vi "Auto Configure DAQ.vi"(8 "error in (no error)":errorcluster, 11 "LockinDAQ":refnum<class "LockinDAQ.lvclass">) -> (0 "error out":errorcluster, 2 "New Ch []":T1[](array[typedef]) {"AI.Coupling" items=["AC"=10045, "DC"=10050, "GND"=10066]}, 3 "LockinDAQ out":refnum<class "LockinDAQ.lvclass">)   [LabVIEW 2016, in "LockinDAQ.lvclass"]
uses:
  LockinDAQ.lvclass
  Typedefs/New Channel Cluster.ctl
  Typedefs/446xAI-enum.ctl
  Typedefs/AI.coupling-enum.ctl
  Typedefs/446xAO-enum.ctl
  Typedefs/AO.config-cluster.ctl
  Typedefs/DAQType-enum.ctl
  Typedefs/AI.config-cluster.ctl
  LockinDAQ.lvclass/LockinDAQ.ctl
  <resource>/objmgr/daqmx.rc
panel:
  # "Device"
  # "AI.Ch"
  # "AI.Range"
  # "AI.Coupling"
  # "AO.Ch"
  # "AO.Range"
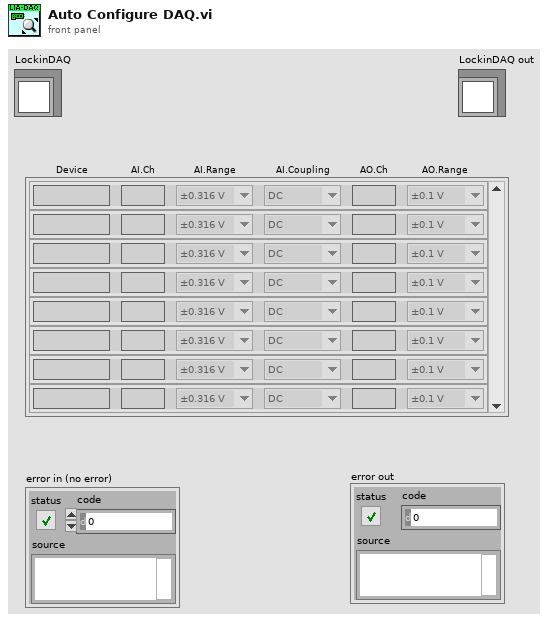
[diagram p1: front panel]
types:
  T1 = typedef "LockinDAQ.lvclass/New Channel Cluster.ctl" = cluster{"Device":string, "AI.Ch":string, "AI.Range":T2, "AI.Coupling":T3, "AO.Ch":string, "AO.Range":T4}
  T2 = typedef "LockinDAQ.lvclass/446xAI-enum.ctl" = enum16{"±0.316 V", "±1.00 V", "±3.16 V", "±10.0 V", "±31.6 V", "±42.4 V"}
  T3 = typedef "LockinDAQ.lvclass/AI.coupling-enum.ctl" = u16
  T4 = typedef "LockinDAQ.lvclass/446xAO-enum.ctl" = enum16{"±0.1 V", "±1.0 V", "±10.0 V"}
  T5 = typedef "LockinDAQ.lvclass/AI.config-cluster.ctl" = cluster{"AI.channels":tag, "AI.Coupling":T3, "AI.Range":T2, "input terminal configuration":i32, "DAQ Type":T6}
  T6 = typedef "LockinDAQ.lvclass/DAQType-enum.ctl" = enum16{"None", "USB 4431", "PXI 446x"}
  T7 = typedef "LockinDAQ.lvclass/AO.config-cluster.ctl" = cluster{"AO.channels":tag, "AO.Range":T4, "output terminal configuration":i32, "DAQ Type":T6}
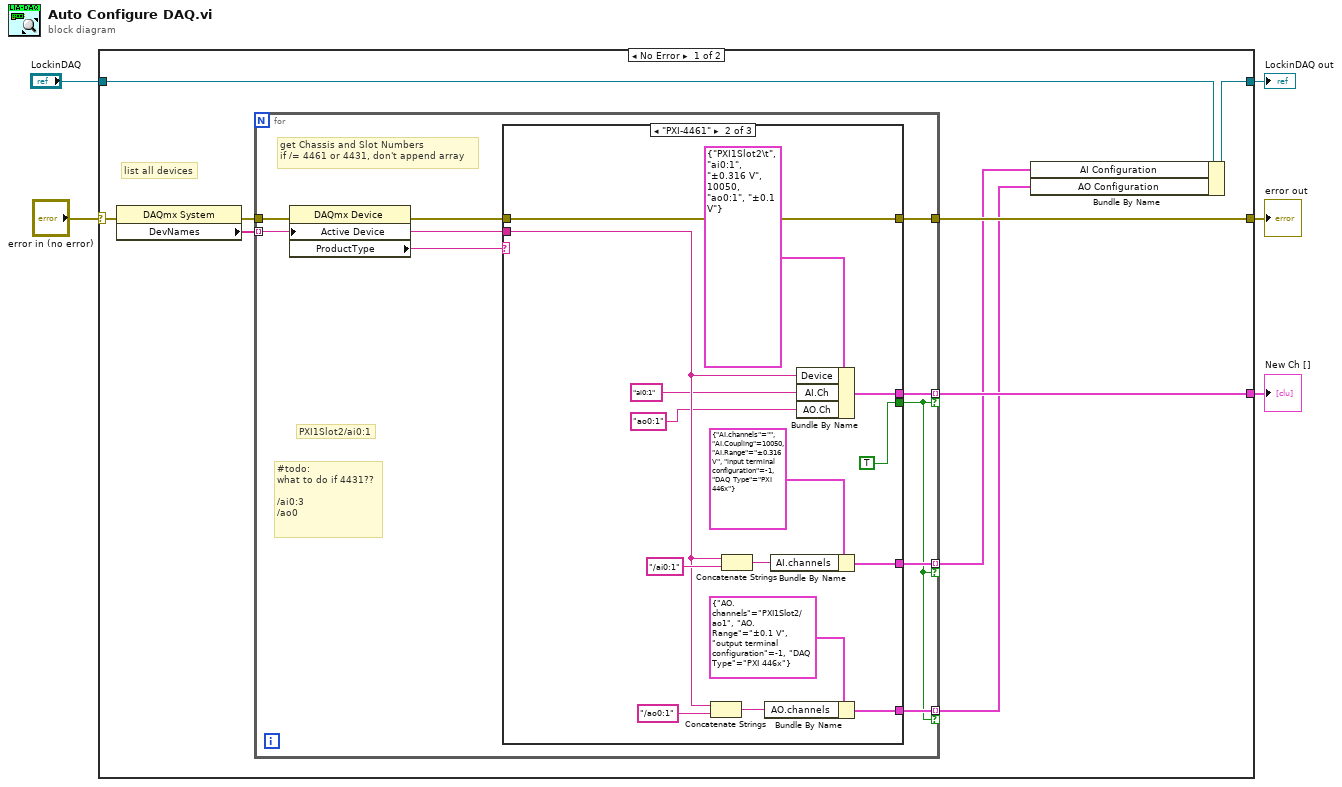
[diagram p0: block diagram]
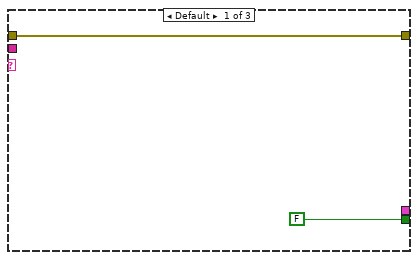
[diagram p2: hidden frame]
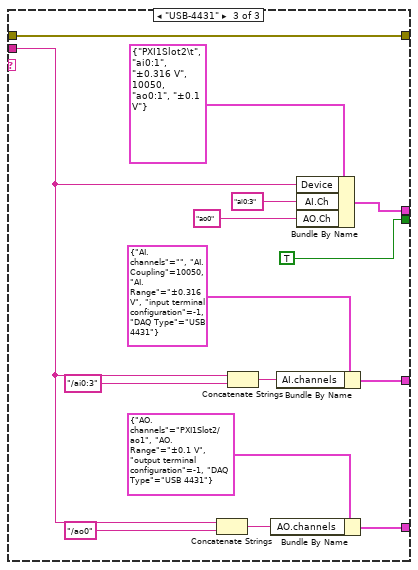
[diagram p3: hidden frame]
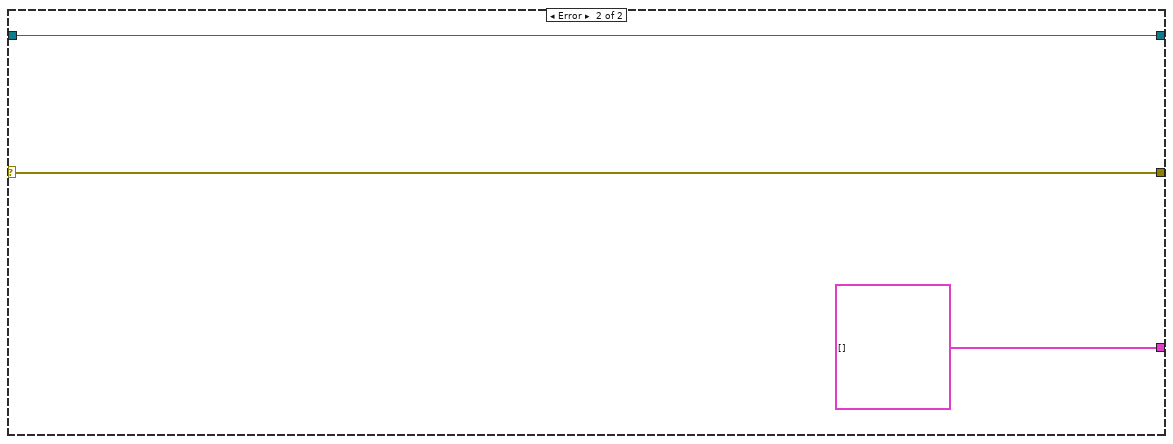
[diagram p4: hidden frame]
diagram:
  n1 = case shown="No Error" "error in (no error)" {
    selector: "error in (no error)" -> [w6 w57]
    tunnel: [w12 T1[] []] -> w5
    tunnel: [w11 w57] -> w4
    tunnel: "LockinDAQ" -> [w10 w58]
    tunnel: [w9 w58] -> w2
    frame No Error {
      # "list all devices"
      n2 = property class="DAQmx System"(error in=w6) -> (error out=w13:errorcluster, "DevNames"=w14:tag[])  [unwired: 1 in, 1 out]
      n3 = for {
        tunnel: w14 -> [w15] mode=indexing
        tunnel: w13 -> [w23]
        tunnel: [w22] -> w12 mode=indexing if=w18
        tunnel: [w16] -> w11
        tunnel: [w21] -> w8 mode=indexing if=w18
        tunnel: [w20] -> w7 mode=indexing if=w18
        # "#todo:\nwhat to do if 4431??\n\n/ai0:3\n/ao0"
        # "PXI1Slot2/ai0:1"
        # "get Chassis and Slot Numbers\nif /= 4461 or 4431, don't append array"
        n4 = property class="DAQmx Device"(error in=w23, "Active Device"=w15) -> (error out=w17:errorcluster, "ProductType"=w19:string)  [unwired: 1 in, 1 out]
        n5 = case shown="\"PXI-4461\"" w19 {
          tunnel: [_ w40 w55] -> w22
          tunnel: [_ w34 w49] -> w21
          tunnel: [_ w33 w48] -> w20
          tunnel: [FALSE TRUE TRUE] -> w18
          tunnel: w17 -> [w24 w29 w41]
          tunnel: [w24 w29 w41] -> w16
          tunnel: w15 -> [_ w28 w44]
          frame Default {
          }
          frame "PXI-4461" {
            n6 = Concatenate Strings(w28, "/ao0:1" ("string")) -> (w37:string)
            n7 = Concatenate Strings(w28, "/ai0:1" ("string")) -> (w31:string)
            n8 = Bundle By Name(cluster=T7 {"AO.channels"="PXI1Slot2/ao1", "AO.Range"=enum."±0.1 V", "output terminal configuration"=-1, "DAQ Type"=enum."PXI 446x"} ("AO.config"), "AO.channels"=w37) -> (w33:T7)
            n9 = Bundle By Name(cluster=T5 {"AI.channels"="", "AI.Coupling"=10050, "AI.Range"=enum."±0.316 V", "input terminal configuration"=-1, "DAQ Type"=enum."PXI 446x"} ("AI.Config"), "AI.channels"=w31) -> (w34:T5)
            n10 = Bundle By Name(cluster=T1 {"Device"="PXI1Slot2\t", "AI.Ch"="ai0:1", "AI.Range"=enum."±0.316 V", "AI.Coupling"=10050, "AO.Ch"="ao0:1", "AO.Range"=enum."±0.1 V"} ("System Cluster"), "Device"=w28, "AI.Ch"="ai0:1" ("string"), "AO.Ch"="ao0:1" ("string")) -> (w40:T1)
          }
          frame "USB-4431" {
            n11 = Concatenate Strings(w44, "/ao0" ("string")) -> (w52:string)
            n12 = Concatenate Strings(w44, "/ai0:3" ("string")) -> (w46:string)
            n13 = Bundle By Name(cluster=T7 {"AO.channels"="PXI1Slot2/ao1", "AO.Range"=enum."±0.1 V", "output terminal configuration"=-1, "DAQ Type"=enum."USB 4431"} ("AO.config"), "AO.channels"=w52) -> (w48:T7)
            n14 = Bundle By Name(cluster=T5 {"AI.channels"="", "AI.Coupling"=10050, "AI.Range"=enum."±0.316 V", "input terminal configuration"=-1, "DAQ Type"=enum."USB 4431"} ("AI.Config"), "AI.channels"=w46) -> (w49:T5)
            n15 = Bundle By Name(cluster=T1 {"Device"="PXI1Slot2\t", "AI.Ch"="ai0:1", "AI.Range"=enum."±0.316 V", "AI.Coupling"=10050, "AO.Ch"="ao0:1", "AO.Range"=enum."±0.1 V"} ("System Cluster"), "Device"=w44, "AI.Ch"="ai0:3", "AO.Ch"="ao0") -> (w55:T1)
          }
        }
      }
      n16 = Bundle By Name(cluster=w10, "AI Configuration"=w8, "AO Configuration"=w7) -> (w9:refnum<class "LockinDAQ.lvclass">)
    }
    frame Error {
    }
  }
  "New Ch []" <- w5
  "error out" <- w4
  "LockinDAQ out" <- w2
